vi "TDMS.ManageHarddrive.vi"(8 "error in":errorcluster, 10 "Remote Path":path=path "d:/testdata/temp", 11 "Results Path":path=path "c:/testdata/temp") -> (0 "error out":errorcluster)   [LabVIEW 2015, in "Analysis.lvlib"]
uses:
  Analysis.lvlib
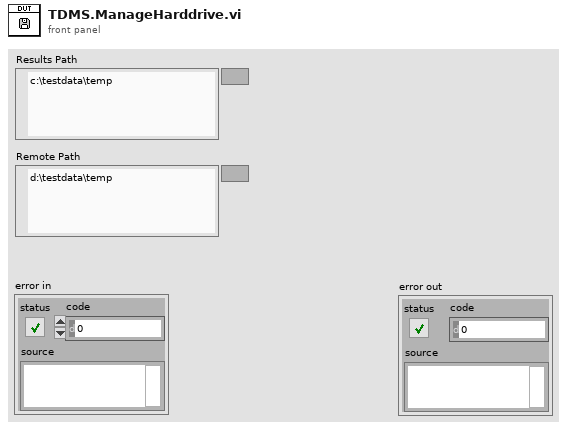
[diagram p1: front panel]
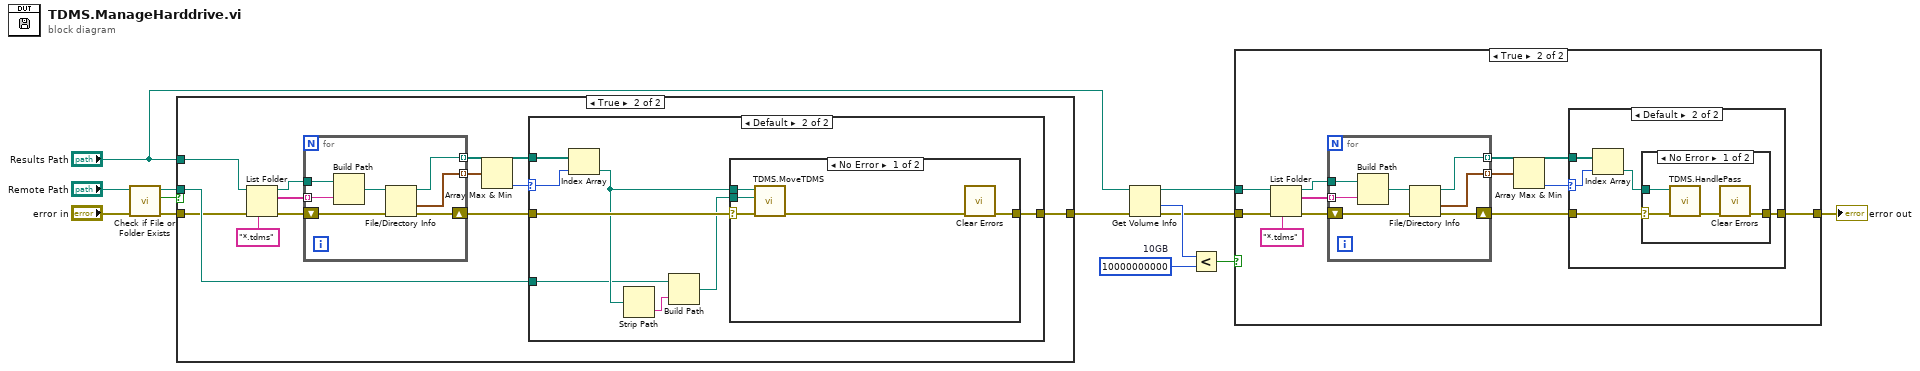
[diagram p0: block diagram]
diagram:
  w6 = i64 10000000000  # 10GB
  n1 = call <vilib>:"Check if File or Folder Exists.vi"("error in (no error)"="error in", "path"="Remote Path") -> ("error out"=w11:errorcluster, "file or folder exists?"=w10:bool, "dup path"=w9:path)  [unwired: 7 in]
  n2 = case shown="True" w10 {
    tunnel: "Results Path" -> [_ w17]
    tunnel: w11 -> [w14 w19]
    tunnel: w9 -> [_ w26]
    tunnel: [w14 w25] -> w8
    frame False {
    }
    frame True {
      n3 = List Folder(path=w17, pattern="*.tdms", error in=w19) -> (path out=w23:path, filenames=w22:string[], error out=w21:errorcluster)  [unwired: 1 in, 1 out]
      n4 = for {
        tunnel: w22 -> [w46] mode=indexing
        tunnel: w23 -> [w47]
        shift-right: [w44] -> w18
        shift-left: w21 -> [w48]
        tunnel: [w43] -> w24 mode=indexing
        tunnel: [w42] -> w16 mode=indexing
        n5 = Build Path(base path=w47, name or relative path=w46) -> (appended path=w45:path)
        n6 = File/Directory Info(path=w45, error in=w48) -> (path out=w42:path, last mod=w43:timestamp, error out=w44:errorcluster)  [unwired: 4 out]
      }
      n7 = Array Max & Min(array=w24) -> (min index (indices)=w15:i32)  [unwired: 3 out]
      n8 = case shown="Default" w15 {
        selector: w15 -> [_ w31]
        tunnel: w26 -> [_ w28]
        tunnel: [w27 w35] -> w25
        tunnel: w18 -> [w27 w34]
        tunnel: w16 -> [_ w33]
        frame -1 {
        }
        frame Default {
          n9 = Index Array(array=w33, index=w31) -> (element=w32:path)
          n10 = Strip Path(path=w32) -> (name=w29:string)  [unwired: 1 out]
          n11 = Build Path(base path=w28, name or relative path=w29) -> (appended path=w30:path)
          n12 = case shown="No Error" w34 {
            selector: w34 -> [w38 w41]
            tunnel: w32 -> [w37 _]
            tunnel: w30 -> [w40 _]
            tunnel: [w39 w41] -> w35
            frame No Error {
              n13 = call "TDMS.MoveTDMS.vi"("error in (no error)"=w38, "Target path"=w40, "Source Path"=w37) -> ("error out"=w36:errorcluster)  [unwired: 8 in]
              n14 = call <vilib>:"Clear Errors.vi"("error in (no error)"=w36) -> ("error out"=w39:errorcluster)  [unwired: 5 in, 1 out]
            }
            frame Error {
            }
          }
        }
      }
    }
  }
  n15 = Get Volume Info(8:w8, 11:"Results Path") -> (0:w4:errorcluster, 1:w7:i64, 3:w2:path)  [unwired: 3 out]
  n16 = Less?(x=w7, y=w6) -> (x < y?=w5:bool)
  n17 = case shown="True" w5 {
    tunnel: w4 -> [w49 w56]
    tunnel: w2 -> [_ w55]
    tunnel: [w49 w52] -> w3
    frame False {
    }
    frame True {
      n18 = List Folder(path=w55, pattern="*.tdms", error in=w56) -> (path out=w57:path, filenames=w58:string[], error out=w59:errorcluster)  [unwired: 1 in, 1 out]
      n19 = for {
        tunnel: w58 -> [w76] mode=indexing
        tunnel: w57 -> [w77]
        shift-right: [w74] -> w51
        shift-left: w59 -> [w78]
        tunnel: [w73] -> w54 mode=indexing
        tunnel: [w72] -> w53 mode=indexing
        n20 = Build Path(base path=w77, name or relative path=w76) -> (appended path=w75:path)
        n21 = File/Directory Info(path=w75, error in=w78) -> (path out=w72:path, last mod=w73:timestamp, error out=w74:errorcluster)  [unwired: 4 out]
      }
      n22 = Array Max & Min(array=w54) -> (min index (indices)=w50:i32)  [unwired: 3 out]
      n23 = case shown="Default" w50 {
        selector: w50 -> [_ w62]
        tunnel: w53 -> [_ w66]
        tunnel: [w61 w64] -> w52
        tunnel: w51 -> [w61 w63]
        frame -1 {
        }
        frame Default {
          n24 = Index Array(array=w66, index=w62) -> (element=w65:path)
          n25 = case shown="No Error" w63 {
            selector: w63 -> [w67 w71]
            tunnel: w65 -> [w70 _]
            tunnel: [w68 w71] -> w64
            frame No Error {
              n26 = call "TDMS.HandlePass.vi"("error in (no error)"=w67, "file path in"=w70) -> ("error out"=w69:errorcluster)  [unwired: 9 in]
              n27 = call <vilib>:"Clear Errors.vi"("error in (no error)"=w69) -> ("error out"=w68:errorcluster)  [unwired: 5 in, 1 out]
            }
            frame Error {
            }
          }
        }
      }
    }
  }
  "error out" <- w3
